vi "Task 2 yg lain.vi"() -> ()   [LabVIEW 2015]
uses:
  Global 17.vi
  Global 12.vi
  Global 15.vi
panel:
  out "Waveform Graph":dynamicdata(graph)
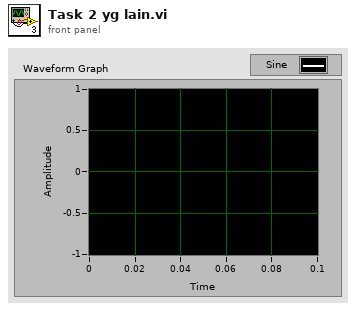
[diagram p1: front panel]
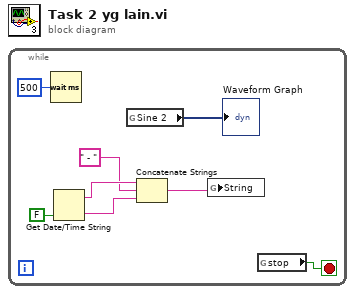
[diagram p0: block diagram]
diagram:
  n1 = while {
    stop <- w6 stop-if-true
    n2 = Wait (ms)(milliseconds to wait=u32 500) -> ()  [unwired: 1 out]
    n3 = Get Date/Time String(want seconds? (F)=FALSE) -> (date string=w4:string, time string=w3:string)  [unwired: 2 in]
    n4 = global read "Global 12.vi" "Sine 2"() -> (→"Waveform Graph":dynamicdata)
    n5 = Concatenate Strings(w4, " - " ("string"), w3) -> (w1:string)
    n6 = global write "Global 17.vi" "String"(w1) -> ()
    n7 = global read "Global 15.vi" "stop"() -> (w6:bool)
  }
